vi "Get Unique List of Property.vi"(6 "System Fields (none)":T1[](array[typedef]), 7 "UserName":string="jimbo", 8 "error in (no error)":errorcluster, 9 "Other Conditions":T4[](array[typedef]), 10 "Value Wildcard String (*)":string, 11 "Display Field Name":string) -> (0 "error out":errorcluster, 1 "Number Found":i32, 2 "Data Returned?":bool, 3 "Unique Name List":string[](array[string]))   [LabVIEW 2011]
uses:
  eSearch Types.ctl
  DataFinder Comparisons.ctl
  Datafinder Query.ctl
  database/Fields/Field Record.ctl
  database/Fields/Field NextItem.ctl
  database/Fields/Field DataTypes.ctl
panel:
  out "Final Query Conditions":T4[](array[typedef])
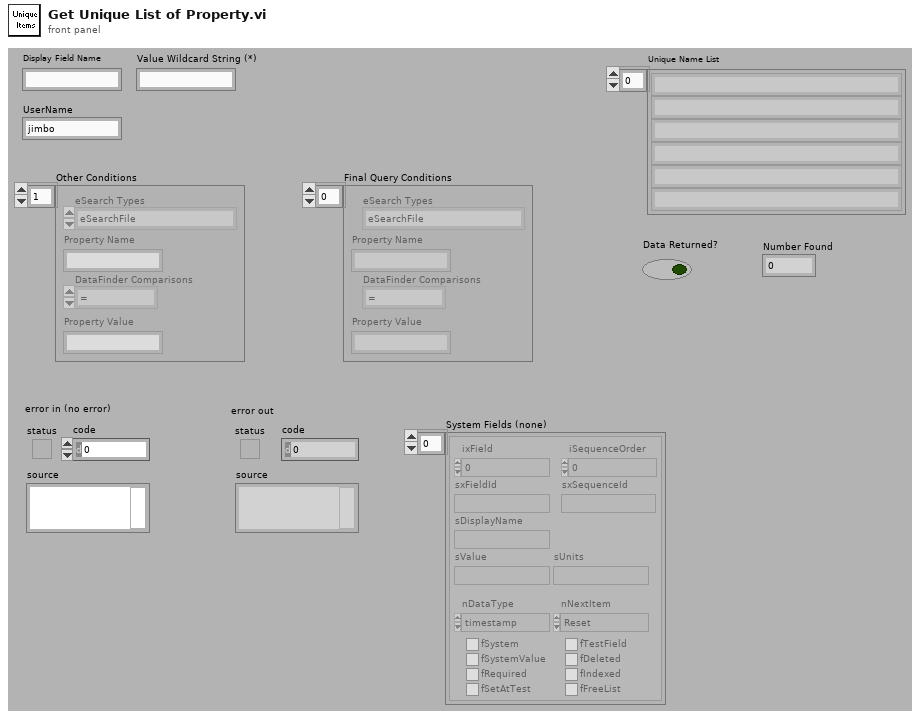
[diagram p1: front panel]
types:
  T1 = typedef "Field Record.ctl" = cluster{"ixField":i32, "iSequenceOrder":i32, "sxFieldId":string, "sxSequenceId":string, "sDisplayName":string, "sValue":string, "sUnits":string, "nDataType":T2, "nNextItem":T3, "fSystem":bool, "fSystemValue":bool, "fRequired":bool, "fSetAtTest":bool, "fTestField":bool, "fDeleted":bool, "fIndexed":bool, "fFreeList":bool}
  T2 = typedef "Field DataTypes.ctl" = enum32{"text", "numeric", "list", "timestamp", "boolean"}
  T3 = typedef "Field NextItem.ctl" = enum32{"Reset", "Retain", "Auto-Increment"}
  T4 = typedef "Datafinder Query.ctl" = cluster{"eSearch Types":T5, "Property Name":string, "DataFinder Comparisons":T6, "Property Value":string}
  T5 = typedef "eSearch Types.ctl" = enum16{"eSearchFile", "eSearchChannelGroup", "eSearchChannel"}
  T6 = typedef "DataFinder Comparisons.ctl" = enum16{"=", "<>", "<", "<=", ">", ">="}
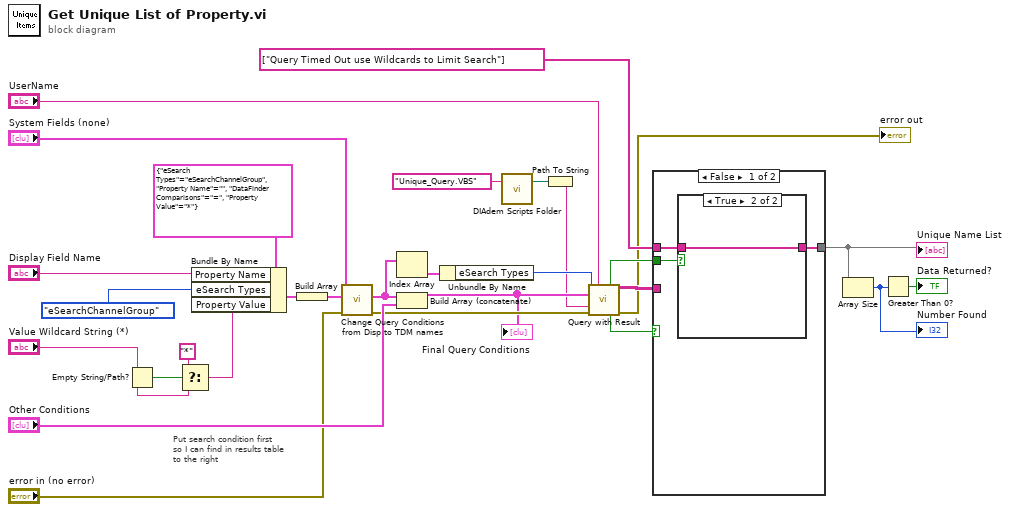
[diagram p0: block diagram]
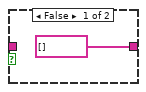
[diagram p2: hidden frame]
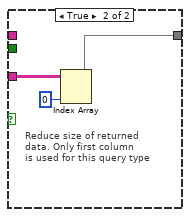
[diagram p3: hidden frame]
diagram:
  # "Put search condition first\nso I can find in results table\nto the right"
  n1 = Empty String/Path?(string/path="Value Wildcard String (*)") -> (empty?=w23:bool)
  n2 = Select(t="*" ("Property Value"), s=w23, f="Value Wildcard String (*)") -> (s? t:f=w20:string)
  n3 = Bundle By Name(cluster=T4 {"eSearch Types"=enum."eSearchChannelGroup", "Property Name"="", "DataFinder Comparisons"=enum."=", "Property Value"="*"} ("Data Finder Parameters"), "Property Name"="Display Field Name", "eSearch Types"=eSearch_Types."eSearchChannelGroup", "Property Value"=w20) -> (w14:T4)
  n4 = Build Array(w14) -> (w17:T4[])
  n5 = call "Change Query Conditions from Disp to TDM names.vi"("error in (no error)"="error in (no error)", "Conditions"=w17, "System Fields (none)"="System Fields (none)") -> ("error out"=w15:errorcluster, "Array"=w16:T4[])  [unwired: 7 out]
  n6 = Index Array(array=w16) -> (element=w9:T4)  [unwired: 1 in]
  n7 = Build Array (concatenate)(w16, "Other Conditions") -> (w13:T4[])
  "Final Query Conditions" <- w13
  n8 = Unbundle By Name(w9) -> ("eSearch Types"=w8:T5)
  n9 = call "DIAdem Scripts Folder.vi"("Relative Path (\"\" - Folder)"="Unique_Query.VBS" ("Query Name.vbs")) -> ("Scripts Folder"=w6:path)  [unwired: 2 out]
  n10 = Path To String(path=w6) -> (string=w4:string)
  n11 = call "Query with Result.vi"("eSearch Type"=w8, "UserName"="UserName", "Search Parameters"=w13, "Query Name.vbs"=w4, "error in (no error)"=w15) -> ("Timed Out?"=w10:bool, "Results"=w12:string[][], "Data Returned?"=w11:bool, "error out"=→"error out":errorcluster)  [unwired: 7 out]
  n12 = case shown="False" w11 {
    tunnel: w12 -> [_ w37]
    tunnel: [w32 w35] -> w27
    tunnel: w10 -> [w31 _]
    tunnel: string[] ["Query Timed Out use Wildcards to Limit Search"] ("Results") -> [w30 _]
    frame False {
      n13 = case shown="True" w31 {
        tunnel: [string[] [] w34] -> w32
        tunnel: w30 -> [_ w34]
        frame False {
        }
        frame True {
        }
      }
    }
    frame True {
      # "Reduce size of returned data. Only first column\nis used for this query type"
      n14 = Index Array(array=w37, index (col)=0 ("disabled index (col)")) -> (element=w35:string[])  [unwired: 1 in]
    }
  }
  "Unique Name List" <- w27
  n15 = Array Size(array=w27) -> (size(s)=w25:i32)
  "Number Found" <- w25
  n16 = Greater Than 0?(x=w25) -> (x > 0?=→"Data Returned?":bool)
